vi "PS Voltage 2 SP Power at Obj.vi"(4 "Switch":bool caption="Power at Obj (F,default)\nPower at interferometer (T)", 5 "SP -> Power Matrix":T1, 6 "Volts S":dbl, 7 "Volts P":dbl) -> (2 "Power S":dbl, 3 "Power P":dbl)   [LabVIEW 2020, in "SignalConverson.lvlib"]
uses:
  SignalConverson.lvlib
  <vilib>/Analysis/Matrix/Datatypes/RealMatrix.ctl
  <vilib>/Analysis/baseanly.llb/A x Vector.vi
  <vilib>/Analysis/NI_AALBase.lvlib
  <vilib>/Analysis/Matrix/NI_Matrix.lvlib
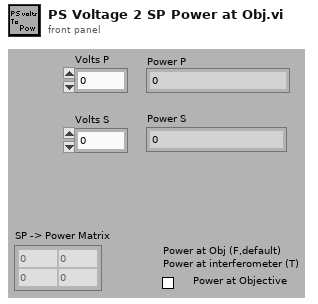
[diagram p1: front panel]
types:
  T1 = typedef "NI_Matrix.lvlib/RealMatrix.ctl" = dbl[][]
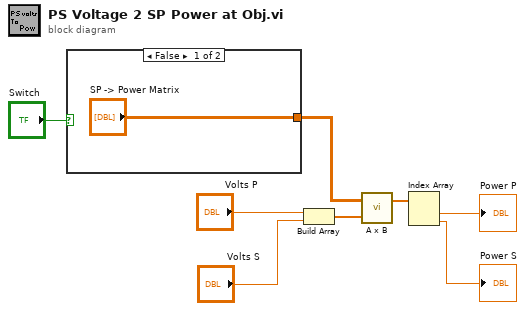
[diagram p0: block diagram]
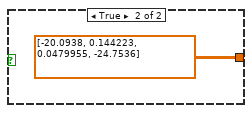
[diagram p2: hidden frame]
diagram:
  n1 = case shown="False" "Switch" {
    tunnel: ["SP -> Power Matrix" T1 [[-20.0938, 0.144223], [0.0479955, -24.7536]] ("SP -> Power Matrix 2")] -> w6
    frame False {
    }
    frame True {
    }
  }
  n2 = Build Array("Volts P", "Volts S") -> (w7:dbl[])
  n3 = call-poly <vilib>:"A x B.vi"("Vector"=w7, "A"=w6) -> ("A x Vector"=w3:dbl[])  [unwired: 1 out]
  n4 = Index Array(array=w3) -> (element #1=→"Power P":dbl, element #2=→"Power S":dbl)  [unwired: 2 in]
